vi "FTW-Test-CSV-Datatypes-Serialize.vi"() -> ()   [LabVIEW 2015]
uses:
  <vilib>/registry/registry.llb/Registry refnum.ctl
  source/Collection/FTW-Collection-KeyValuePair.ctl
  source/actor/Message/Request/FTW-Message-IncomingRequest.lvclass
  source/Reflection/FTW-Reflection-Types.ctl
  <vilib>/FTP/ftp0.llb/FTP Session.ctl
  <vilib>/httpClient/ClientHandle.ctl
  <vilib>/FTP/NI_FTP.lvlib
  <vilib>/httpClient/LabVIEWHTTPClient.lvlib
panel:
  in  "Timestamp Format":string="%^<%Y-%m-%dT%H:%M:%S%3uZ>T"
  in  "Real Format":string="%#.6f"
  in  "String Quotes":bool
  out "Strings":string[](array[string])
  out "Errors":errorcluster[](array[cluster])
  in  "DynamicData":dynamicdata(waveform)
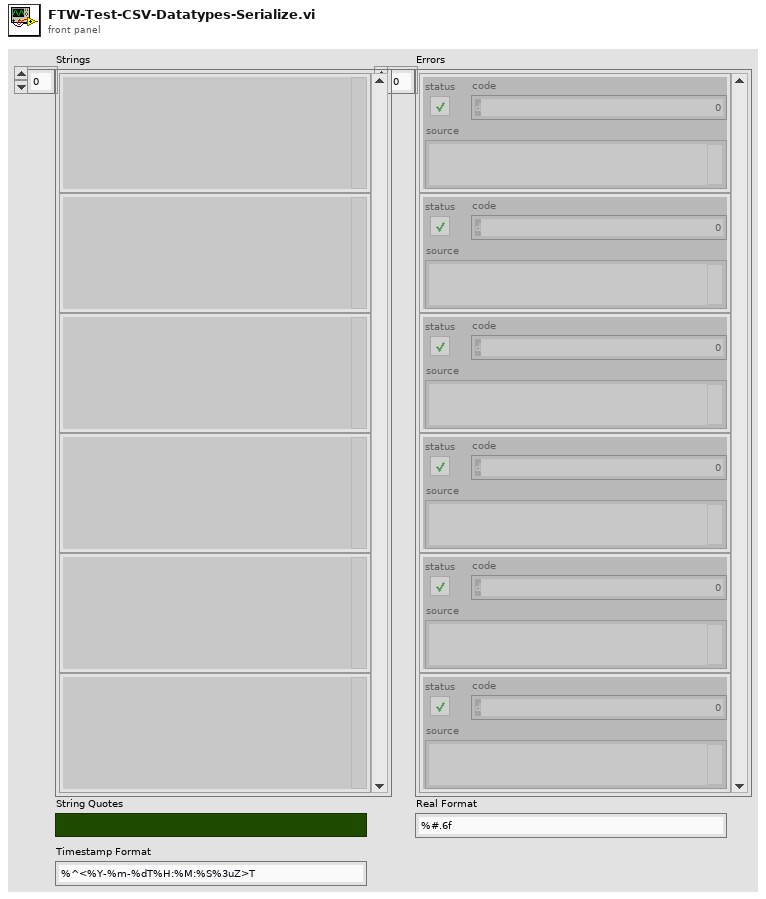
[diagram p1: front panel]
types:
  T1 = typedef "LabVIEWHTTPClient.lvlib/ClientHandle.ctl" = refnum<k1>
  T2 = typedef "NI_FTP.lvlib/FTP Session.ctl" = refnum<k5>
  T3 = typedef "FTW-Reflection-Types.ctl" = enum16{"Unknown", "Void", "Array", "Cluster", "LVObject", "Boolean", "I8", "I16", "I32", "I64", "U8", "U16", "U32", "U64", "SGL", "DBL", "EXT", "CSG", "CDB", "CXT", "FXP", "EnumU8", "EnumU16", "EnumU32", "EnumU64", "SGLwithUnit", "DBLwithUnit", "EXTwithUnit", "CSGwithUnit", "CDBwithUnit", "CXTwithUnit", "String", "Path", "Picture", "Tag", "LVVariant", "Timestamp", "WaveformI8", "WaveformI16", "WaveformI32", "WaveformI64", "WaveformU8", "WaveformU16", "WaveformU32", "WaveformU64", "WaveformSGL", "WaveformDBL", "WaveformEXT", "WaveformCSG", "WaveformCDB", "WaveformCXT", "WaveformDigital", "WaveformUnknownType", "DigitalData", "DynamicData", "ExternalData", "FileByteStream", "TDMStream", "dotNET", "ActiveX", "VIServerReference", "VIReference", "ApplicationInstance", "Menu", "ConnectionDataSocket", "ConnectionVISA", "ConnectionBluetooth", "ConnectionIrDA", "ConnectionTCP", "ConnectionUDP", "ConnectionHTTPClient", "ConnectionFTP", "Occurrence", "Notifier", "Queue", "Rendezvous", "Semaphore", "RTFIFO", "EventPublisher", "EventRegistration", "EventCallback", "DataValueReference", "GenericClass", "GenericClassTag", "GenericClassDeepCopy", "GenericClassFlattened", "GenericClassTagFlattened", "GenericReferenceType", "WindowsRegistry", "OverloadedDatalogRef", "ReferenceUnknownType"}
  T4 = typedef "FTW-Collection-KeyValuePair.ctl" = cluster{"Key":string, "Value":string}
  T5 = typedef "Registry refnum.ctl" = refnum<k1>
  T6 = typedef "Rendezvous RefNum" = refnum<k1>
  T7 = typedef "Semaphore RefNum" = refnum<k1>
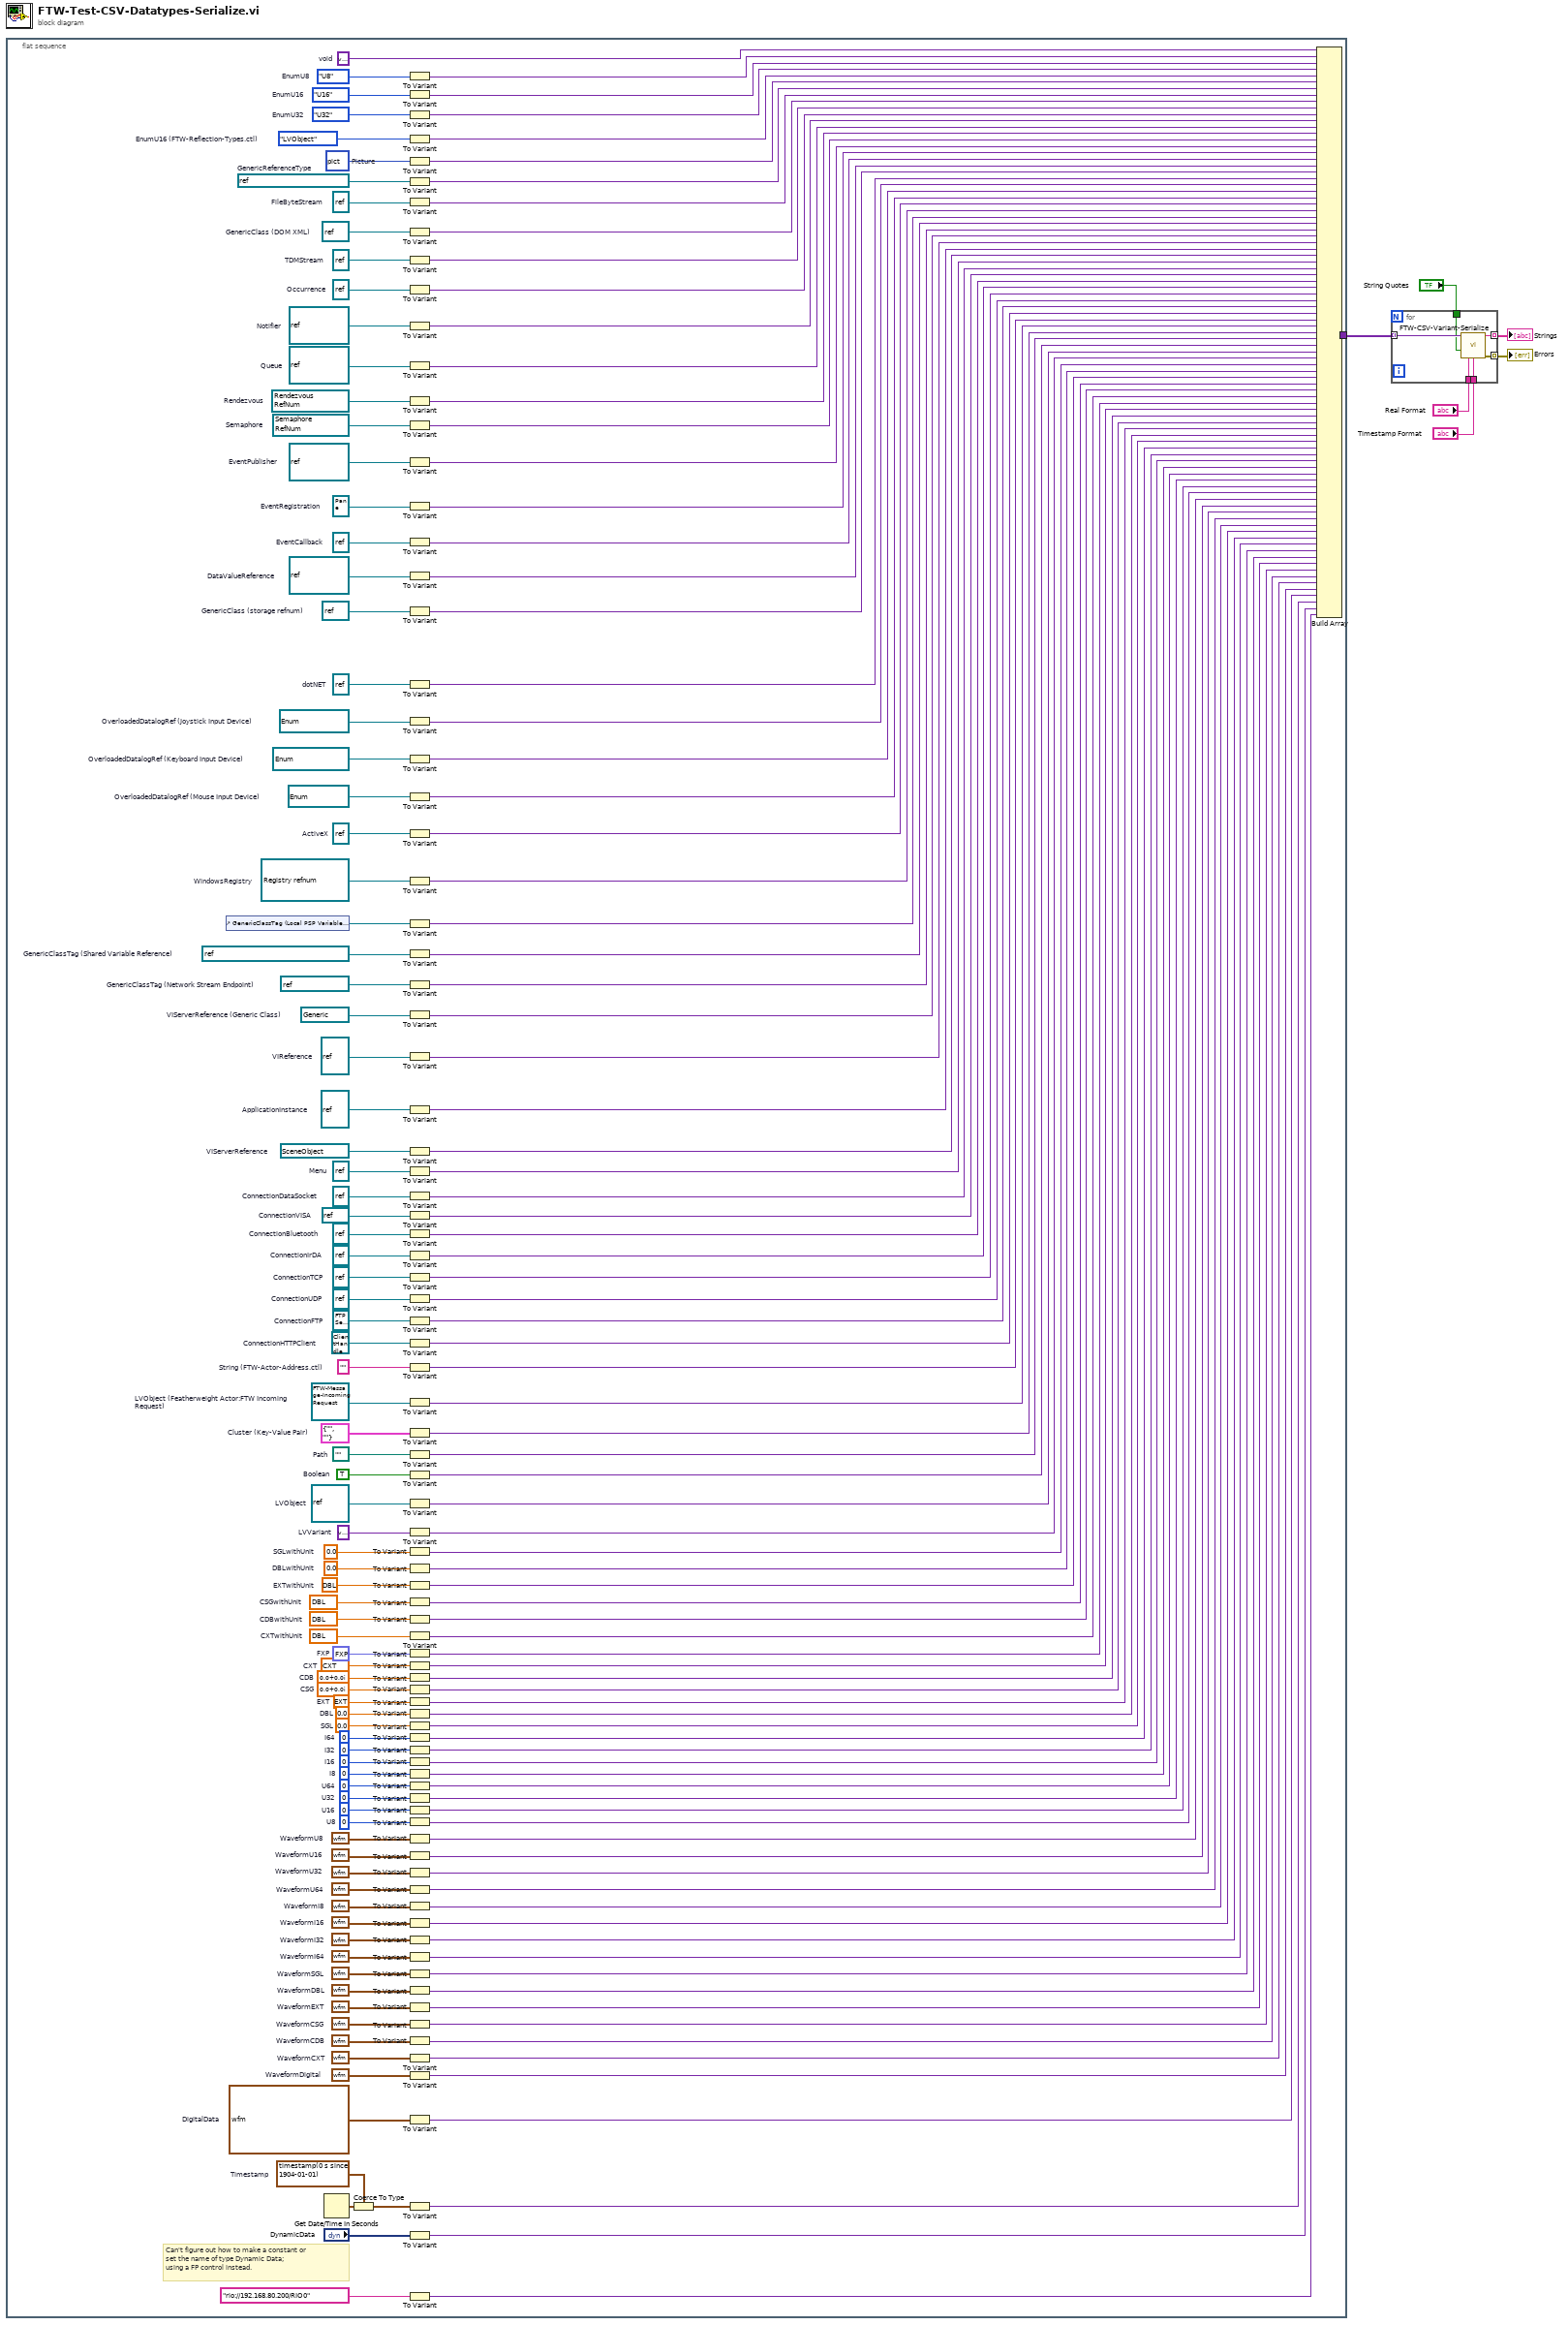
[diagram p0: block diagram]
diagram:
  n1 = flat-sequence {
    tunnel: [w185] -> w6
    frame #0 {
      w13 = digitalwaveform {"t0"=timestamp(0 s since 1904-01-01), "dt"=0.0, "Y"={"transitions"=[], "data"=[]}}  # WaveformDigital
      w14 = waveform(cxt) {"t0"=timestamp(0 s since 1904-01-01), "dt"=1.0, "Y"=[]}  # WaveformCXT
      w15 = waveform(cdb) {"t0"=timestamp(0 s since 1904-01-01), "dt"=1.0, "Y"=[]}  # WaveformCDB
      w16 = waveform(csg) {"t0"=timestamp(0 s since 1904-01-01), "dt"=1.0, "Y"=[]}  # WaveformCSG
      w17 = waveform(ext) {"t0"=timestamp(0 s since 1904-01-01), "dt"=1.0, "Y"=[]}  # WaveformEXT
      w18 = waveform(dbl) {"t0"=timestamp(0 s since 1904-01-01), "dt"=1.0, "Y"=[]}  # WaveformDBL
      w19 = waveform(sgl) {"t0"=timestamp(0 s since 1904-01-01), "dt"=1.0, "Y"=[]}  # WaveformSGL
      w20 = waveform(i64) {"t0"=timestamp(0 s since 1904-01-01), "dt"=1.0, "Y"=[]}  # WaveformI64
      w21 = waveform(i32) {"t0"=timestamp(0 s since 1904-01-01), "dt"=1.0, "Y"=[]}  # WaveformI32
      w22 = waveform(i16) {"t0"=timestamp(0 s since 1904-01-01), "dt"=1.0, "Y"=[]}  # WaveformI16
      w26 = waveform(i8) {"t0"=timestamp(0 s since 1904-01-01), "dt"=1.0, "Y"=[]}  # WaveformI8
      w27 = waveform(u64) {"t0"=timestamp(0 s since 1904-01-01), "dt"=1.0, "Y"=[]}  # WaveformU64
      w25 = waveform(u32) {"t0"=timestamp(0 s since 1904-01-01), "dt"=1.0, "Y"=[]}  # WaveformU32
      w24 = waveform(u16) {"t0"=timestamp(0 s since 1904-01-01), "dt"=1.0, "Y"=[]}  # WaveformU16
      w23 = waveform(u8) {"t0"=timestamp(0 s since 1904-01-01), "dt"=1.0, "Y"=[]}  # WaveformU8
      w28 = variant  # void
      w112 = refnum<k31> refnum  # ConnectionBluetooth
      w117 = T1 refnum  # ConnectionHTTPClient
      w70 = T2 refnum  # ConnectionFTP
      w79 = enum32{"U32"}."U32"  # EnumU32
      w78 = enum16{"U16"}."U16"  # EnumU16
      w77 = enum8{"U8"}."U8"  # EnumU8
      w116 = TRUE  # Boolean
      w121 = path ""  # Path
      w80 = FTW-Reflection-Types."LVObject"  # EnumU16 (FTW-Reflection-Types.ctl)
      w119 = refnum<class "FTW-Message-IncomingRequest.lvclass"> refnum  # LVObject (Featherweight Actor:FTW Incoming Request)
      w89 = refnum<event-registration> refnum  # EventRegistration
      w120 = T4 {"Key"="", "Value"=""}  # Cluster (Key-Value Pair)
      w118 = ""  # String (FTW-Actor-Address.ctl)
      w115 = refnum<k16> refnum  # ConnectionUDP
      w114 = refnum<k5> refnum  # ConnectionTCP
      w110 = refnum<k13> refnum  # ConnectionDataSocket
      w109 = refnum<k9> refnum  # Menu
      w93 = refnum<data-value> refnum  # DataValueReference
      w113 = refnum<k19> refnum  # ConnectionIrDA
      w81 = picture data[5B]  # Picture
      w108 = refnum<vi> refnum  # VIServerReference
      w106 = refnum<vi> refnum  # ApplicationInstance
      w107 = refnum<vi> refnum  # VIReference
      w105 = refnum<vi> refnum  # VIServerReference (Generic Class)
      w104 = refnum<k21> "localhost"  # GenericClassTag (Network Stream Endpoint)
      w94 = refnum<k27> refnum  # EventCallback
      w90 = refnum<user-event> refnum  # EventPublisher
      w86 = refnum<k4> refnum  # Occurrence
      w87 = refnum<queue> refnum  # Queue
      w88 = refnum<notifier> refnum  # Notifier
      w103 = refnum<k21> "ni.var.psp://localhost/System"  # GenericClassTag (Shared Variable Reference)
      w100 = refnum<k7> refnum  # ActiveX
      w95 = refnum<k24> refnum  # dotNET
      w96 = refnum<k20> refnum  # GenericClass (storage refnum)
      w85 = refnum<k34> refnum  # TDMStream
      w82 = refnum<k0> refnum  # GenericReferenceType
      w111 = refnum<visa-resource-name> refnum  # ConnectionVISA
      w84 = refnum<k20> refnum  # GenericClass (DOM XML)
      w83 = refnum<file> refnum  # FileByteStream
      w123 = refnum<class> refnum  # LVObject
      w125 = variant  # LVVariant
      w137 = cxt[unit] 0.0+0.0i  # CXTwithUnit
      w136 = cdb[unit] 0.0+0.0i  # CDBwithUnit
      w135 = csg[unit] 0.0+0.0i  # CSGwithUnit
      w134 = ext[unit] 0.0  # EXTwithUnit
      w133 = dbl[unit] 0.0  # DBLwithUnit
      w132 = sgl[unit] 0.0  # SGLwithUnit
      w184 = timestamp(0 s since 1904-01-01)  # Timestamp
      w154 = cxt 0.0+0.0i  # CXT
      w155 = cdb 0.0+0.0i  # CDB
      w156 = csg 0.0+0.0i  # CSG
      w153 = fxp<+/-,64,1024> 0.0  # FXP
      w157 = ext 0.0  # EXT
      w158 = 0.0  # DBL
      w159 = sgl 0.0  # SGL
      w160 = i64 0  # I64
      w161 = 0  # I32
      w162 = i16 0  # I16
      w163 = i8 0  # I8
      w164 = u64 0  # U64
      w165 = u32 0  # U32
      w166 = u16 0  # U16
      w167 = u8 0  # U8
      w186 = digitaldata {"transitions"=[], "data"=[]}  # DigitalData
      w101 = T5 refnum  # WindowsRegistry
      w99 = refnum<k1> refnum items=["MOUSE"]  # OverloadedDatalogRef (Mouse Input Device)
      w97 = refnum<k1> refnum items=["KEYBOARD"]  # OverloadedDatalogRef (Keyboard Input Device)
      w98 = refnum<k1> refnum items=["JOYSTICK"]  # OverloadedDatalogRef (Joystick Input Device)
      w92 = T6 refnum items=["rendezvous"]  # Rendezvous
      w91 = T7 refnum items=["semaphore"]  # Semaphore
      # "Can't figure out how to make a constant or\nset the name of type Dynamic Data;\nusing a FP control instead."
      n2 = control-ref of="GenericClassTag (Local PSP Variable Engine)"() -> (w102:refnum<k21>)
      n3 = Get Date/Time In Seconds() -> (seconds since 1Jan1904=w7:timestamp)
      n4 = Coerce To Type(0:w7, 1:w184) -> (2:w8:timestamp)
      n5 = To Variant(anything=w77) -> (Variant=w30:variant)
      n6 = To Variant(anything=w78) -> (Variant=w31:variant)
      n7 = To Variant(anything=w79) -> (Variant=w32:variant)
      n8 = To Variant(anything=w80) -> (Variant=w33:variant)
      n9 = To Variant(anything=w81) -> (Variant=w34:variant)
      n10 = To Variant(anything=w82) -> (Variant=w35:variant)
      n11 = To Variant(anything=w83) -> (Variant=w36:variant)
      n12 = To Variant(anything=w84) -> (Variant=w37:variant)
      n13 = To Variant(anything=w85) -> (Variant=w38:variant)
      n14 = To Variant(anything=w86) -> (Variant=w39:variant)
      n15 = To Variant(anything=w88) -> (Variant=w40:variant)
      n16 = To Variant(anything=w87) -> (Variant=w41:variant)
      n17 = To Variant(anything=w92) -> (Variant=w42:variant)
      n18 = To Variant(anything=w91) -> (Variant=w43:variant)
      n19 = To Variant(anything=w90) -> (Variant=w44:variant)
      n20 = To Variant(anything=w89) -> (Variant=w45:variant)
      n21 = To Variant(anything=w94) -> (Variant=w46:variant)
      n22 = To Variant(anything=w93) -> (Variant=w47:variant)
      n23 = To Variant(anything=w96) -> (Variant=w48:variant)
      n24 = To Variant(anything=w95) -> (Variant=w49:variant)
      n25 = To Variant(anything=w98) -> (Variant=w50:variant)
      n26 = To Variant(anything=w97) -> (Variant=w51:variant)
      n27 = To Variant(anything=w99) -> (Variant=w52:variant)
      n28 = To Variant(anything=w100) -> (Variant=w53:variant)
      n29 = To Variant(anything=w101) -> (Variant=w54:variant)
      n30 = To Variant(anything=w102) -> (Variant=w55:variant)
      n31 = To Variant(anything=w103) -> (Variant=w56:variant)
      n32 = To Variant(anything=w104) -> (Variant=w57:variant)
      n33 = To Variant(anything=w105) -> (Variant=w58:variant)
      n34 = To Variant(anything=w107) -> (Variant=w59:variant)
      n35 = To Variant(anything=w106) -> (Variant=w60:variant)
      n36 = To Variant(anything=w108) -> (Variant=w61:variant)
      n37 = To Variant(anything=w109) -> (Variant=w62:variant)
      n38 = To Variant(anything=w110) -> (Variant=w63:variant)
      n39 = To Variant(anything=w111) -> (Variant=w64:variant)
      n40 = To Variant(anything=w112) -> (Variant=w65:variant)
      n41 = To Variant(anything=w113) -> (Variant=w66:variant)
      n42 = To Variant(anything=w114) -> (Variant=w67:variant)
      n43 = To Variant(anything=w115) -> (Variant=w68:variant)
      n44 = To Variant(anything=w70) -> (Variant=w69:variant)
      n45 = To Variant(anything=w117) -> (Variant=w71:variant)
      n46 = To Variant(anything=w118) -> (Variant=w72:variant)
      n47 = To Variant(anything=w119) -> (Variant=w73:variant)
      n48 = To Variant(anything=w120) -> (Variant=w74:variant)
      n49 = To Variant(anything=w121) -> (Variant=w75:variant)
      n50 = To Variant(anything=w116) -> (Variant=w76:variant)
      n51 = To Variant(anything=w123) -> (Variant=w122:variant)
      n52 = To Variant(anything=w125) -> (Variant=w124:variant)
      n53 = To Variant(anything=w132) -> (Variant=w126:variant)
      n54 = To Variant(anything=w133) -> (Variant=w127:variant)
      n55 = To Variant(anything=w134) -> (Variant=w128:variant)
      n56 = To Variant(anything=w135) -> (Variant=w129:variant)
      n57 = To Variant(anything=w136) -> (Variant=w130:variant)
      n58 = To Variant(anything=w137) -> (Variant=w131:variant)
      n59 = To Variant(anything=w153) -> (Variant=w138:variant)
      n60 = To Variant(anything=w154) -> (Variant=w139:variant)
      n61 = To Variant(anything=w155) -> (Variant=w140:variant)
      n62 = To Variant(anything=w156) -> (Variant=w141:variant)
      n63 = To Variant(anything=w157) -> (Variant=w142:variant)
      n64 = To Variant(anything=w158) -> (Variant=w143:variant)
      n65 = To Variant(anything=w159) -> (Variant=w144:variant)
      n66 = To Variant(anything=w160) -> (Variant=w145:variant)
      n67 = To Variant(anything=w161) -> (Variant=w146:variant)
      n68 = To Variant(anything=w162) -> (Variant=w147:variant)
      n69 = To Variant(anything=w163) -> (Variant=w148:variant)
      n70 = To Variant(anything=w164) -> (Variant=w149:variant)
      n71 = To Variant(anything=w165) -> (Variant=w150:variant)
      n72 = To Variant(anything=w166) -> (Variant=w151:variant)
      n73 = To Variant(anything=w167) -> (Variant=w152:variant)
      n74 = To Variant(anything=w23) -> (Variant=w183:variant)
      n75 = To Variant(anything=w24) -> (Variant=w182:variant)
      n76 = To Variant(anything=w25) -> (Variant=w181:variant)
      n77 = To Variant(anything=w27) -> (Variant=w180:variant)
      n78 = To Variant(anything=w26) -> (Variant=w179:variant)
      n79 = To Variant(anything=w22) -> (Variant=w178:variant)
      n80 = To Variant(anything=w21) -> (Variant=w177:variant)
      n81 = To Variant(anything=w20) -> (Variant=w176:variant)
      n82 = To Variant(anything=w19) -> (Variant=w175:variant)
      n83 = To Variant(anything=w18) -> (Variant=w174:variant)
      n84 = To Variant(anything=w17) -> (Variant=w173:variant)
      n85 = To Variant(anything=w16) -> (Variant=w172:variant)
      n86 = To Variant(anything=w15) -> (Variant=w171:variant)
      n87 = To Variant(anything=w14) -> (Variant=w170:variant)
      n88 = To Variant(anything=w13) -> (Variant=w169:variant)
      n89 = To Variant(anything=w186) -> (Variant=w168:variant)
      n90 = To Variant(anything=w8) -> (Variant=w29:variant)
      n91 = To Variant(anything="DynamicData") -> (Variant=w12:variant)
      n92 = To Variant(anything=tag "rio://192.168.80.200/RIO0" ("RIO Device")) -> (Variant=w9:variant)
      n93 = Build Array(w28, w30, w31, w32, w33, w34, w35, w36, w37, w38, w39, w40, w41, w42, w43, w44, w45, w46, w47, w48, w49, w50, w51, w52, w53, w54, w55, w56, w57, w58, w59, w60, w61, w62, w63, w64, w65, w66, w67, w68, w69, w71, w72, w73, w74, w75, w76, w122, w124, w126, w127, w128, w129, w130, w131, w138, w139, w140, w141, w142, w143, w144, w145, w146, w147, w148, w149, w150, w151, w152, w183, w182, w181, w180, w179, w178, w177, w176, w175, w174, w173, w172, w171, w170, w169, w168, w29, w12, w9) -> (w185:variant[])
    }
  }
  n94 = for {
    tunnel: w6 -> [w192] mode=indexing
    tunnel: [w191] -> w5 mode=indexing
    tunnel: [w190] -> w4 mode=indexing
    tunnel: "String Quotes" -> [w189]
    tunnel: "Real Format" -> [w188]
    tunnel: "Timestamp Format" -> [w187]
    n95 = call "FTW-CSV-Variant-Serialize.vi"("Variant"=w192, "String Quotes"=w189, "Real Format"=w188, "Timestamp Format"=w187) -> ("CSV String"=w190:string, "error out"=w191:errorcluster)  [unwired: 10 in]
  }
  "Errors" <- w5
  "Strings" <- w4
